vi "IntakeStateMachine.vi"(8 "SlowButton":bool, 9 "FastButton":bool, 10 "Joystick":dbl(slide) scale=-1.0..1.0, 11 "Cluster":T1={"OutakeSpeed"=0.4, "OutakeSpeed Fast"=1.0, "Intake Sens"=1.2, "OutakeSens"=0.7} {"OutakeSpeed Fast" format="%#_13g"; "OutakeSpeed" format="%#_13g"}) -> (2 "Left Intake":dbl format="%#_13g", 3 "Right Intake":dbl)   [LabVIEW 2017]
uses:
  IntakeStates.ctl
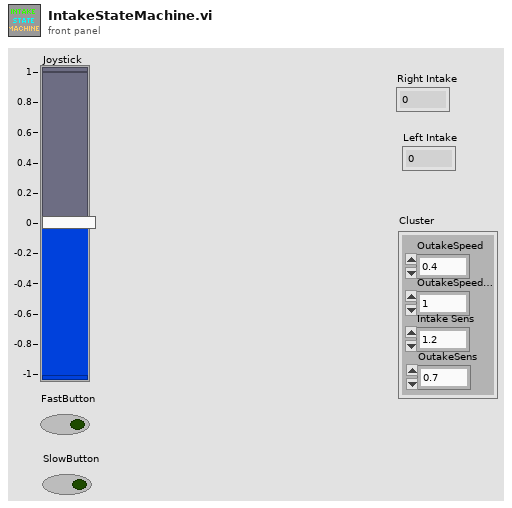
[diagram p1: front panel]
types:
  T1 = cluster{"OutakeSpeed":dbl, "OutakeSpeed Fast":dbl, "Intake Sens":dbl, "OutakeSens":dbl}
  T2 = typedef "IntakeStates.ctl" = enum16{"Intake Manual", "Outtake Manual", "Fast Auto Outake", "Slow Auto Outake", "Dislodging"}
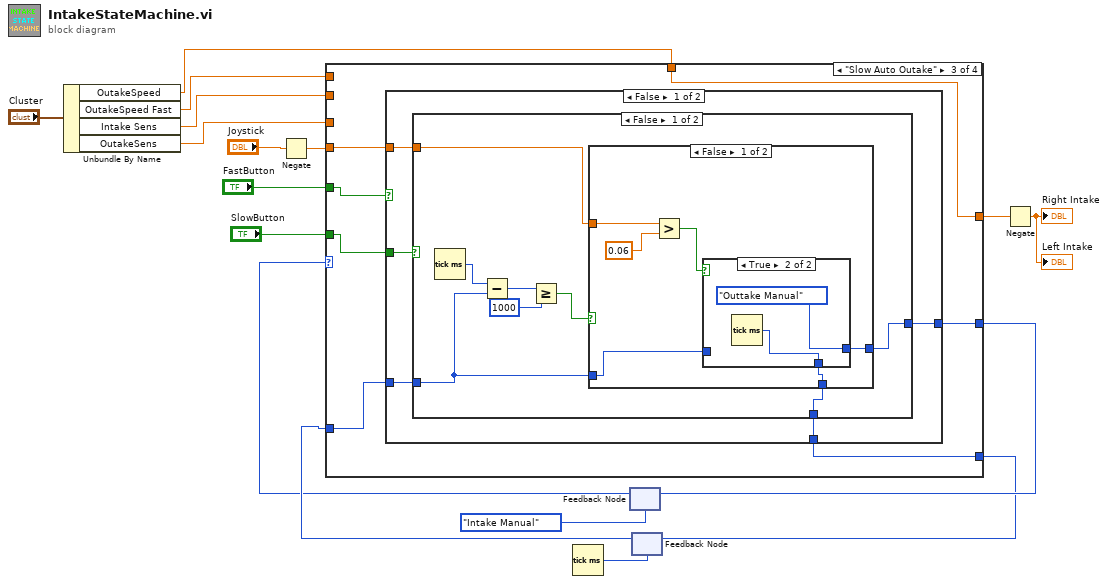
[diagram p0: block diagram]
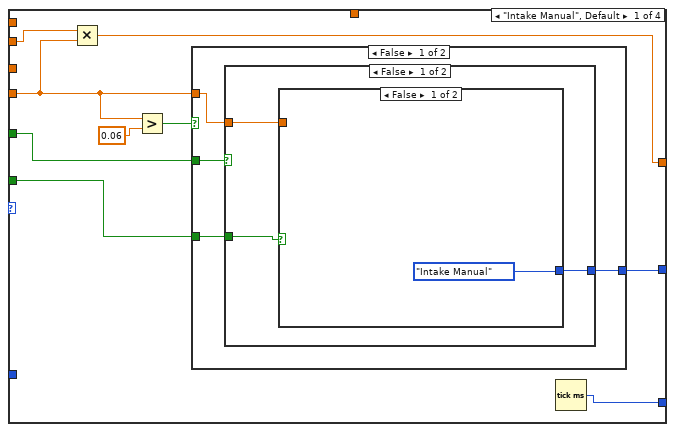
[diagram p2: hidden frame]
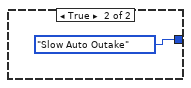
[diagram p3: hidden frame]
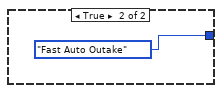
[diagram p4: hidden frame]
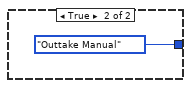
[diagram p5: hidden frame]
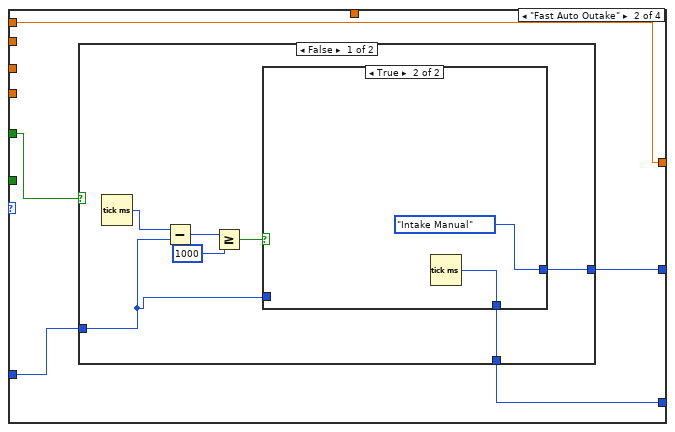
[diagram p6: hidden frame]
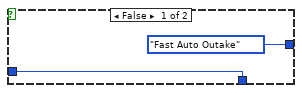
[diagram p7: hidden frame]
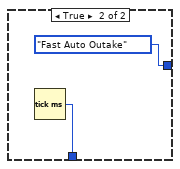
[diagram p8: hidden frame]
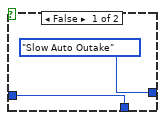
[diagram p9: hidden frame]
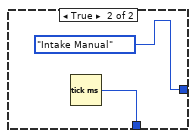
[diagram p10: hidden frame]
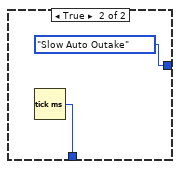
[diagram p11: hidden frame]
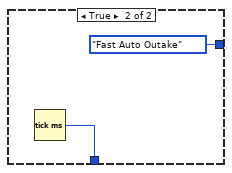
[diagram p12: hidden frame]
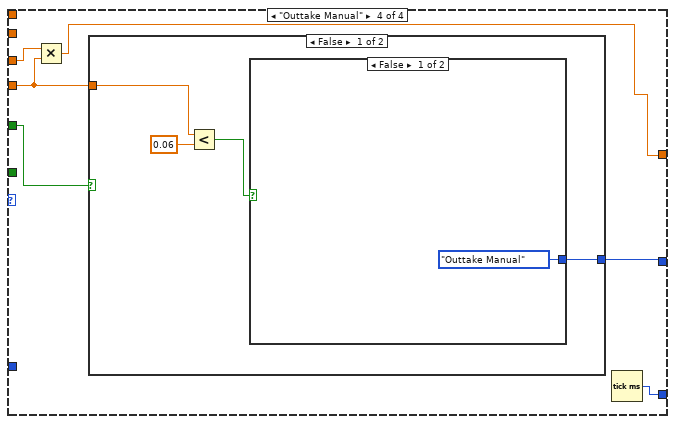
[diagram p13: hidden frame]
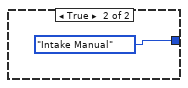
[diagram p14: hidden frame]
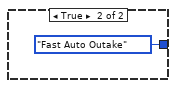
[diagram p15: hidden frame]
diagram:
  n1 = Unbundle By Name("Cluster") -> ("OutakeSpeed"=w7:dbl, "OutakeSpeed Fast"=w8:dbl, "Intake Sens"=w5:dbl, "OutakeSens"=w6:dbl)
  n2 = Negate(x="Joystick") -> (-x=w2:dbl)
  n3 = Tick Count (ms)() -> (millisecond timer value=w13:u32)
  n4 = feedback #1(IntakeStates."Intake Manual" ("States")) -> (w4:T2)
  n5 = feedback #2(w13) -> (w12:u32)
  n6 = case shown="\"Slow Auto Outake\"" w4 {
    tunnel: [w19 w38 w58 w94] -> w10
    tunnel: [w24 w40 w61 w95] -> w16
    tunnel: w2 -> [w20 _ w56 w92]
    tunnel: "FastButton" -> [w23 w42 w57 w96]
    tunnel: "SlowButton" -> [w22 _ w59 _]
    tunnel: w7 -> [_ _ w58 _]
    tunnel: w12 -> [_ w39 w60 _]
    tunnel: [w21 w41 w62 w97] -> w11
    tunnel: w8 -> [_ w38 _ _]
    tunnel: w6 -> [_ _ _ w93]
    tunnel: w5 -> [w18 _ _ _]
    frame "Intake Manual", Default {
      n7 = Multiply(x=w18, y=w20) -> (x*y=w19:dbl)
      n8 = Greater?(x=w20, y=0.06) -> (0:w25:bool)
      n9 = case shown="False" w25 {
        tunnel: [w29 IntakeStates."Outtake Manual" ("States")] -> w24
        tunnel: w20 -> [w27 _]
        tunnel: w23 -> [w30 _]
        tunnel: w22 -> [w28 _]
        frame False {
          n10 = case shown="False" w30 {
            tunnel: [w32 IntakeStates."Fast Auto Outake" ("States")] -> w29
            tunnel: w28 -> [w33 _]
            tunnel: w27 -> [w31 _]
            frame False {
              n11 = case shown="False" w33 {
                tunnel: [IntakeStates."Intake Manual" ("States") IntakeStates."Slow Auto Outake" ("States")] -> w32
                tunnel: w31 -> [_ _]
                frame False {
                }
                frame True {
                }
              }
            }
            frame True {
            }
          }
        }
        frame True {
        }
      }
      n12 = Tick Count (ms)() -> (millisecond timer value=w21:u32)
    }
    frame "Fast Auto Outake" {
      n13 = case shown="False" w42 {
        tunnel: [w44 w55] -> w41
        tunnel: [w45 IntakeStates."Fast Auto Outake" ("States")] -> w40
        tunnel: w39 -> [w43 _]
        frame False {
          n14 = Tick Count (ms)() -> (millisecond timer value=w49:u32)
          n15 = Subtract(x=w49, y=w43) -> (x-y=w48:u32)
          n16 = Greater Or Equal?(x=w48, y=u32 1000) -> (x >= y?=w46:bool)
          n17 = case shown="True" w46 {
            tunnel: [IntakeStates."Fast Auto Outake" ("States") IntakeStates."Intake Manual" ("States")] -> w45
            tunnel: [w50 w52] -> w44
            tunnel: w43 -> [w50 _]
            frame False {
            }
            frame True {
              n18 = Tick Count (ms)() -> (millisecond timer value=w52:u32)
            }
          }
        }
        frame True {
          n19 = Tick Count (ms)() -> (millisecond timer value=w55:u32)
        }
      }
    }
    frame "Slow Auto Outake" {
      n20 = case shown="False" w57 {
        tunnel: [w67 w90] -> w62
        tunnel: [w66 IntakeStates."Fast Auto Outake" ("States")] -> w61
        tunnel: w60 -> [w65 _]
        tunnel: w59 -> [w64 _]
        tunnel: w56 -> [w63 _]
        frame False {
          n21 = case shown="False" w64 {
            tunnel: [w70 w89] -> w67
            tunnel: [w71 IntakeStates."Slow Auto Outake" ("States")] -> w66
            tunnel: w65 -> [w69 _]
            tunnel: w63 -> [w68 _]
            frame False {
              n22 = Tick Count (ms)() -> (millisecond timer value=w75:u32)
              n23 = Subtract(x=w75, y=w69) -> (x-y=w74:u32)
              n24 = Greater Or Equal?(x=w74, y=u32 1000) -> (x >= y?=w72:bool)
              n25 = case shown="False" w72 {
                tunnel: [w81 IntakeStates."Intake Manual" ("States")] -> w71
                tunnel: [w76 w86] -> w70
                tunnel: w69 -> [w78 _]
                tunnel: w68 -> [w79 _]
                frame False {
                  n26 = Greater?(x=w79, y=0.06) -> (0:w77:bool)
                  n27 = case shown="True" w77 {
                    tunnel: [IntakeStates."Slow Auto Outake" ("States") IntakeStates."Outtake Manual" ("States")] -> w81
                    tunnel: w78 -> [w82 _]
                    tunnel: [w82 w84] -> w76
                    frame False {
                    }
                    frame True {
                      n28 = Tick Count (ms)() -> (millisecond timer value=w84:u32)
                    }
                  }
                }
                frame True {
                  n29 = Tick Count (ms)() -> (millisecond timer value=w86:u32)
                }
              }
            }
            frame True {
              n30 = Tick Count (ms)() -> (millisecond timer value=w89:u32)
            }
          }
        }
        frame True {
          n31 = Tick Count (ms)() -> (millisecond timer value=w90:u32)
        }
      }
    }
    frame "Outtake Manual" {
      n32 = Multiply(x=w93, y=w92) -> (x*y=w94:dbl)
      n33 = case shown="False" w96 {
        tunnel: [w99 IntakeStates."Fast Auto Outake" ("States")] -> w95
        tunnel: w92 -> [w101 _]
        frame False {
          n34 = Less?(x=w101, y=0.06) -> (x < y?=w98:bool)
          n35 = case shown="False" w98 {
            tunnel: [IntakeStates."Outtake Manual" ("States") IntakeStates."Intake Manual" ("States")] -> w99
            frame False {
            }
            frame True {
            }
          }
        }
        frame True {
        }
      }
      n36 = Tick Count (ms)() -> (millisecond timer value=w97:u32)
    }
  }
  n37 = feedback-in #1(w16) -> ()
  n38 = feedback-in #2(w11) -> ()
  n39 = Negate(x=w10) -> (-x=→"Right Intake" →"Left Intake":dbl)
